vi "gl_Triggering globals.vi"() -> ()   [LabVIEW 2013]
uses:
  Typedefs/Triggered tasks cluster.ctl
panel:
  out "Triggered tasks cluster":T1
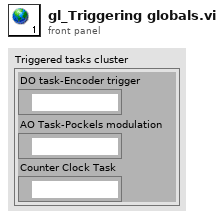
[diagram p1: front panel]
types:
  T1 = typedef "Triggered tasks cluster.ctl" = cluster{"DO task-Encoder trigger":refnum<k21>, "AO Task-Pockels modulation":refnum<k21>, "Counter Clock Task":refnum<k21>}
diagram:
